vi "PicoScope3000aAdvancedTriggerSettingsV2.vi"(0 "error in":errorcluster, 1 "handle in":i16, 3 "Trigger Conditions":T6 {"Condition Logic" items=["AND", "OR", "XOR"]}, 4 "Trigger Delay":u32, 5 "Auto Trigger (ms)":i32=1000, 6 "Channel A Trigger Properties":T3={"thresholdUpper"=0, "thresholdUpperHysteresis"=5, "thresholdLower"=0, "thresholdLowerHysteresis"=5, "Threshold Mode"=0, "Direction"=2, "Available"=FALSE} {"Direction" items=["Above / Inside", "Below / Outside", "Rising / Enter", "Falling / Exit", "Rising or Falling / Enter or Exit", "Above Lower", "Below Lower", "Rising Lower", "Falling Lower", "Positive Runt", "Negative Runt"]; "Threshold Mode" items=["Level", "Window"]}, 7 "Channel D Trigger Properties":T3={"thresholdUpper"=0, "thresholdUpperHysteresis"=0, "thresholdLower"=0, "thresholdLowerHysteresis"=0, "Threshold Mode"=0, "Direction"=2, "Available"=FALSE} {"Direction" items=["Above / Inside", "Below / Outside", "Rising / Enter", "Falling / Exit", "Rising or Falling / Enter or Exit", "Above Lower", "Below Lower", "Rising Lower", "Falling Lower", "Positive Runt", "Negative Runt"]; "Threshold Mode" items=["Level", "Window"]}, 8 "Channel B Trigger Properties":T3={"thresholdUpper"=0, "thresholdUpperHysteresis"=0, "thresholdLower"=0, "thresholdLowerHysteresis"=0, "Threshold Mode"=0, "Direction"=2, "Available"=FALSE} {"Direction" items=["Above / Inside", "Below / Outside", "Rising / Enter", "Falling / Exit", "Rising or Falling / Enter or Exit", "Above Lower", "Below Lower", "Rising Lower", "Falling Lower", "Positive Runt", "Negative Runt"]; "Threshold Mode" items=["Level", "Window"]}, 10 "Digital Port  0":T2 {"Direction Channel 7" items=["Don't Care", "Low", "High", "Rising", "Falling"]; "Direction Channel 6" items=["Don't Care", "Low", "High", "Rising", "Falling"]; "Direction Channel 5" items=["Don't Care", "Low", "High", "Rising", "Falling"]; "Direction Channel 4" items=["Don't Care", "Low", "High", "Rising", "Falling"]; "Direction Channel 3" items=["Don't Care", "Low", "High", "Rising", "Falling"]; "Direction Channel 2" items=["Don't Care", "Low", "High", "Rising", "Falling"]; "Direction Channel 1" items=["Don't Care", "Low", "High", "Rising", "Falling"]; "Direction Channel 0" items=["Don't Care", "Low", "High", "Rising", "Falling"]}, 11 "Ext. Trigger Properties":T3={"thresholdUpper"=0, "thresholdUpperHysteresis"=0, "thresholdLower"=0, "thresholdLowerHysteresis"=0, "Threshold Mode"=0, "Direction"=2, "Available"=FALSE} {"Direction" items=["Above / Inside", "Below / Outside", "Rising / Enter", "Falling / Exit", "Rising or Falling / Enter or Exit", "Above Lower", "Below Lower", "Rising Lower", "Falling Lower", "Positive Runt", "Negative Runt"]; "Threshold Mode" items=["Level", "Window"]}, 12 "Digital Port  1":T1 {"Direction Channel 15" items=["Don't Care", "Low", "High", "Rising", "Falling"]; "Direction Channel 14" items=["Don't Care", "Low", "High", "Rising", "Falling"]; "Direction Channel 13" items=["Don't Care", "Low", "High", "Rising", "Falling"]; "Direction Channel 12" items=["Don't Care", "Low", "High", "Rising", "Falling"]; "Direction Channel 11" items=["Don't Care", "Low", "High", "Rising", "Falling"]; "Direction Channel 10" items=["Don't Care", "Low", "High", "Rising", "Falling"]; "Direction Channel 9" items=["Don't Care", "Low", "High", "Rising", "Falling"]; "Direction Channel 8" items=["Don't Care", "Low", "High", "Rising", "Falling"]}, 13 "Aux. Trigger Properties":T3={"thresholdUpper"=0, "thresholdUpperHysteresis"=0, "thresholdLower"=0, "thresholdLowerHysteresis"=0, "Threshold Mode"=0, "Direction"=2, "Available"=FALSE} {"Direction" items=["Above / Inside", "Below / Outside", "Rising / Enter", "Falling / Exit", "Rising or Falling / Enter or Exit", "Above Lower", "Below Lower", "Rising Lower", "Falling Lower", "Positive Runt", "Negative Runt"]; "Threshold Mode" items=["Level", "Window"]}, 16 "Channel C Trigger Properties":T3={"thresholdUpper"=0, "thresholdUpperHysteresis"=0, "thresholdLower"=0, "thresholdLowerHysteresis"=0, "Threshold Mode"=0, "Direction"=2, "Available"=FALSE} {"Direction" items=["Above / Inside", "Below / Outside", "Rising / Enter", "Falling / Exit", "Rising or Falling / Enter or Exit", "Above Lower", "Below Lower", "Rising Lower", "Falling Lower", "Positive Runt", "Negative Runt"]; "Threshold Mode" items=["Level", "Window"]}, 18 "Pulse Width Qualifier Conditions":T5 {"Condition Logic" items=["AND", "OR", "XOR"]}, 19 "Pulse Width Qualifier Settings":T4={"Direction"=2, "Lower Limit"=0, "Upper Limit"=0, "Pulse Width Type"=0} {"Pulse Width Type" items=["None", "Less Than", "Greater Than", "In Range", "Out of Range"]; "Direction" items=["Rising"=2, "Falling"=3]}) -> (14 "error out":errorcluster, 15 "handle out":i16)   [LabVIEW 2010]
doc: "This VI is an interface for the advanced trigger features of the oscilloscope (a simple trigger can be set using PicoScope3000aSettings.vi, in which case it is not necessary to use this VI)."
uses:
  ps3000a.dll
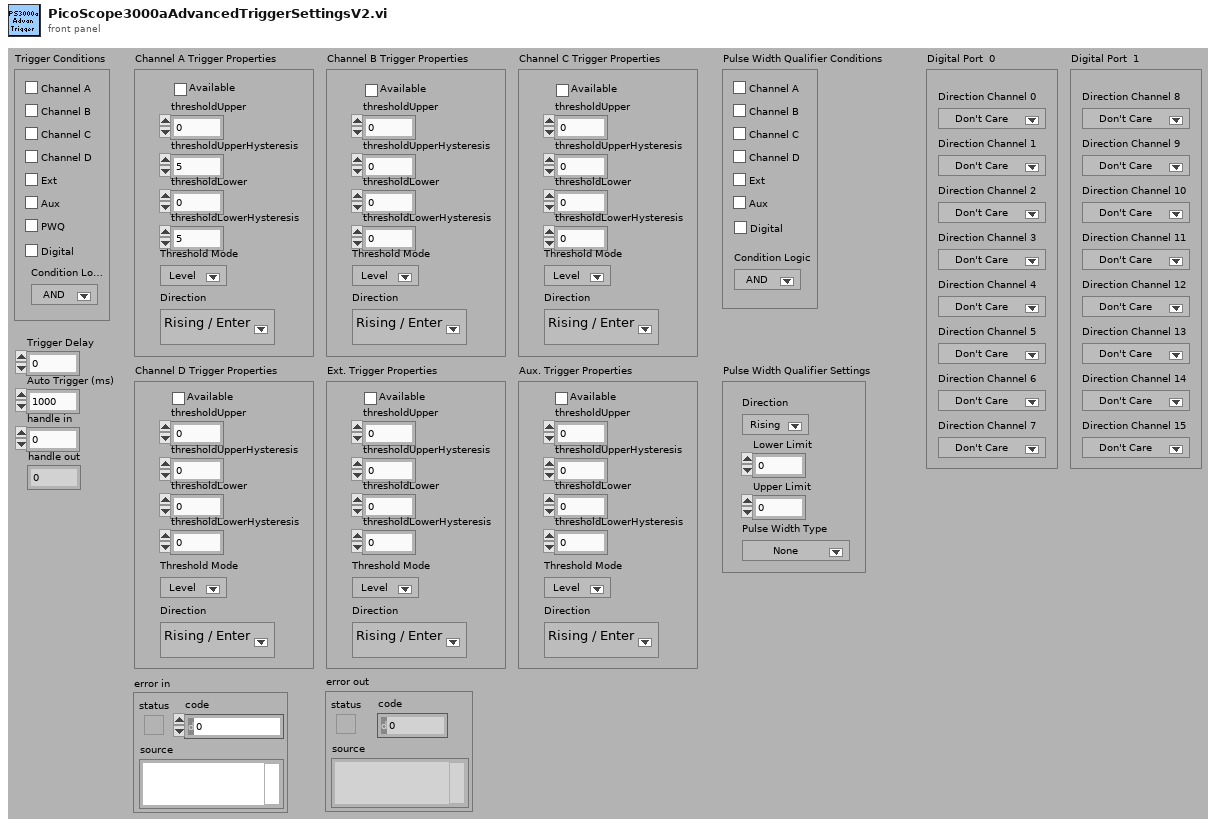
[diagram p1: front panel]
types:
  T1 = cluster{"Direction Channel 8":u16, "Direction Channel 9":u16, "Direction Channel 10":u16, "Direction Channel 11":u16, "Direction Channel 12":u16, "Direction Channel 13":u16, "Direction Channel 14":u16, "Direction Channel 15":u16}
  T2 = cluster{"Direction Channel 0":u16, "Direction Channel 1":u16, "Direction Channel 2":u16, "Direction Channel 3":u16, "Direction Channel 4":u16, "Direction Channel 5":u16, "Direction Channel 6":u16, "Direction Channel 7":u16}
  T3 = cluster{"thresholdUpper":i16, "thresholdUpperHysteresis":u16, "thresholdLower":i16, "thresholdLowerHysteresis":u16, "Threshold Mode":i32, "Direction":i32, "Available":bool}
  T4 = cluster{"Direction":u32, "Lower Limit":u32, "Upper Limit":u32, "Pulse Width Type":u32}
  T5 = cluster{"Channel A":bool, "Channel B":bool, "Channel C":bool, "Channel D":bool, "Aux":bool, "Condition Logic":u16, "Ext":bool, "Digital":bool}
  T6 = cluster{"Channel A":bool, "Channel B":bool, "Channel C":bool, "Channel D":bool, "Aux":bool, "PWQ":bool, "Condition Logic":u16, "Ext":bool, "Digital":bool}
  T7 = cluster{"thresholdUpper":i16, "thresholdUpperHysteresis":u16, "thresholdLower":i16, "thresholdLowerHysteresis":u16, "Threshold Mode":i32, "Direction":i32, "Available":bool}[]
  T8 = cluster{"[0]":u32, "[1]":u32, "[2]":u32, "[3]":u32, "[4]":u32, "[5]":u32, "[6]":u32, "[7]":u32, "[8]":u32}
  T9 = cluster{"status":bool, "code":u32, "source":string}
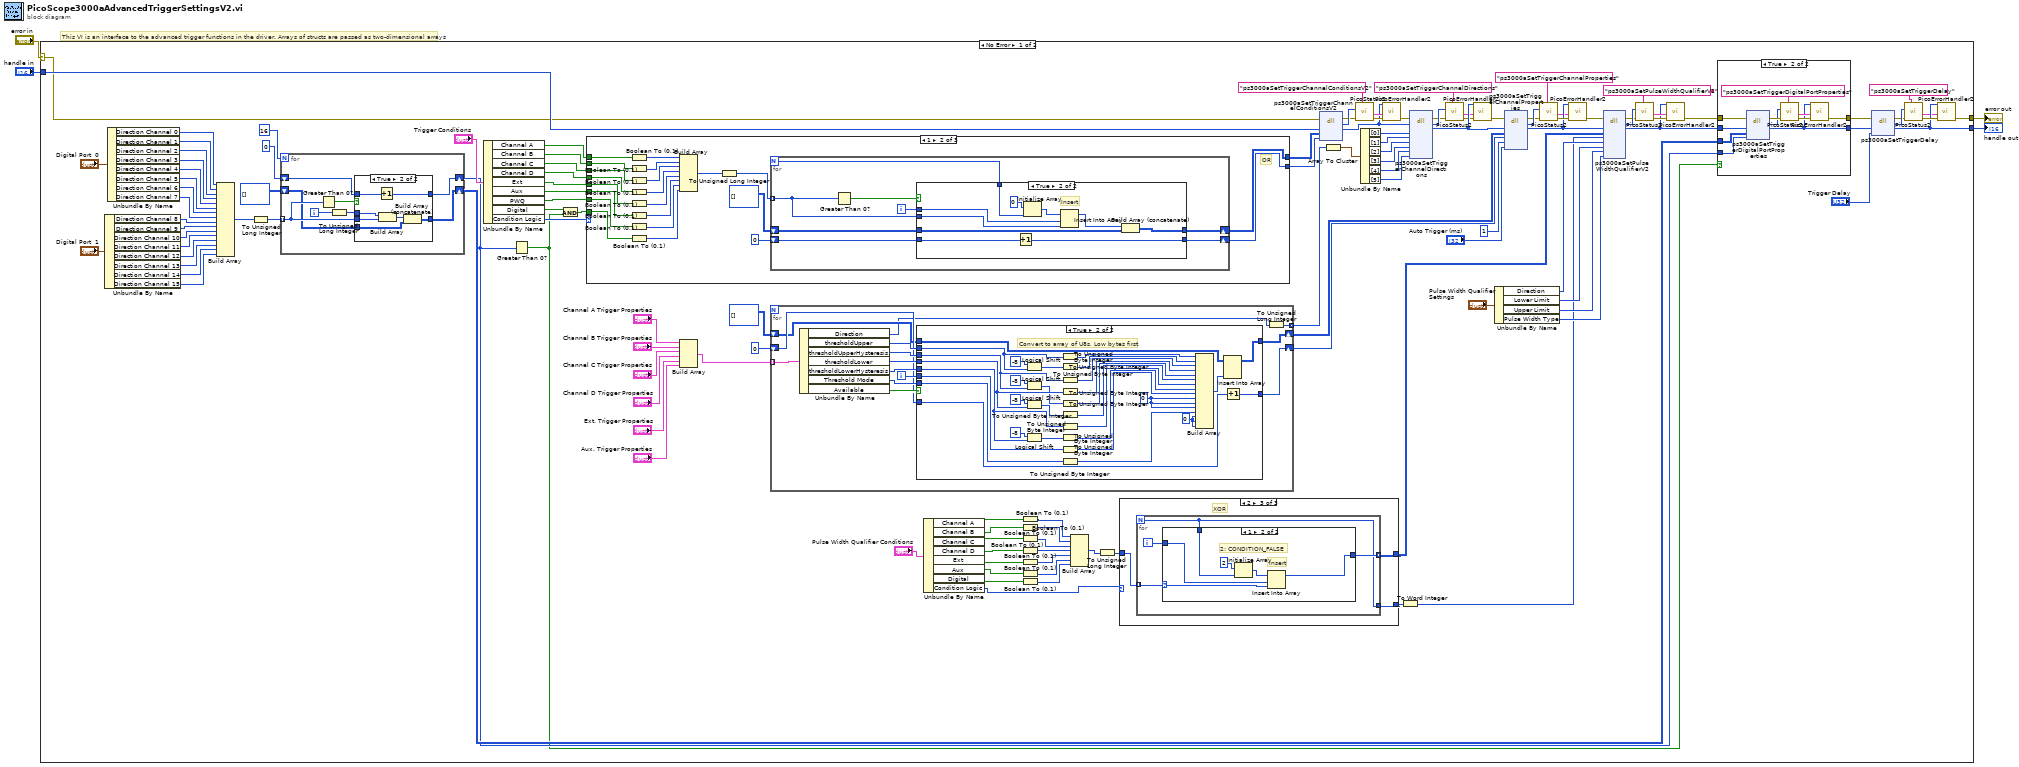
[diagram p0: block diagram]
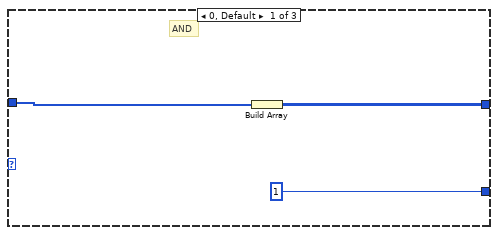
[diagram p2: hidden frame]
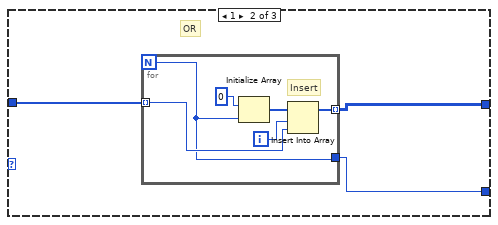
[diagram p3: hidden frame]
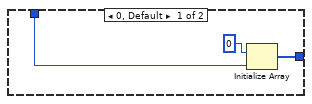
[diagram p4: hidden frame]
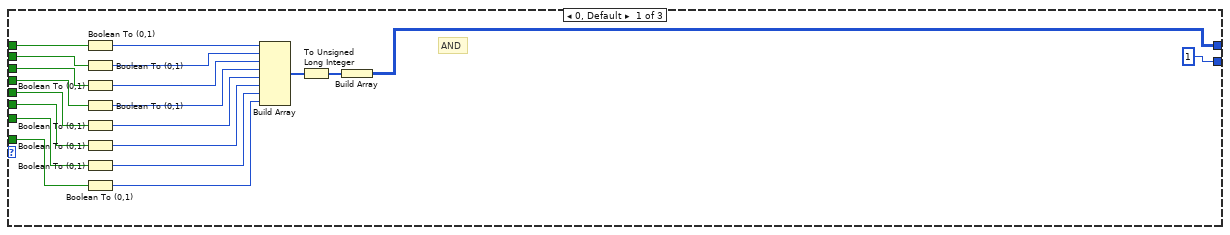
[diagram p8: hidden frame]
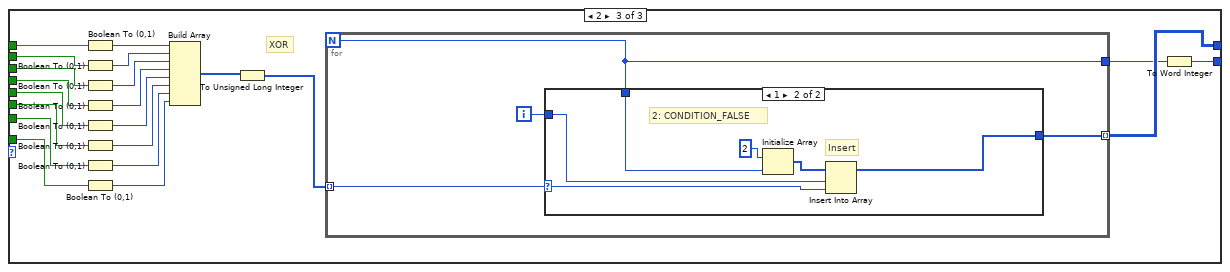
[diagram p10: hidden frame]
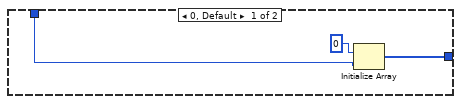
[diagram p11: hidden frame]
diagram:
  # "This VI is an interface to the advanced trigger functions in the driver. Arrays of structs are passed as two-dimensional arrays"
  n1 = case shown="No Error" "error in" {
    selector: "error in" -> [w100 w332]
    tunnel: "handle in" -> [w104 w333]
    tunnel: [w43 w333] -> w2
    tunnel: [w44 w332] -> w1
    frame No Error {
      n2 = Unbundle By Name("Digital Port  1") -> ("Direction Channel 8"=w66:u16, "Direction Channel 9"=w65:u16, "Direction Channel 10"=w64:u16, "Direction Channel 11"=w63:u16, "Direction Channel 12"=w62:u16, "Direction Channel 13"=w61:u16, "Direction Channel 14"=w60:u16, "Direction Channel 15"=w59:u16)
      n3 = Unbundle By Name("Digital Port  0") -> ("Direction Channel 0"=w78:u16, "Direction Channel 1"=w77:u16, "Direction Channel 2"=w76:u16, "Direction Channel 3"=w75:u16, "Direction Channel 4"=w74:u16, "Direction Channel 5"=w73:u16, "Direction Channel 6"=w72:u16, "Direction Channel 7"=w71:u16)
      n4 = Build Array(w78, w77, w76, w75, w74, w73, w72, w71, w66, w65, w64, w63, w62, w61, w60, w59) -> (w38:u16[])
      n5 = To Unsigned Long Integer(number=w38) -> (unsigned 32bit integer=w39:u32[])
      n6 = for {
        N: 16 -> [_]
        tunnel: w39 -> [w178] mode=indexing
        shift-right: [w177] -> w56
        shift-left: u32[][] [] -> [w176]
        shift-right: [w175] -> w53
        shift-left: i16 0 -> [w174]
        i -> [w172]
        n7 = Greater Than 0?(x=w178) -> (x > 0?=w179:bool)
        n8 = To Unsigned Long Integer(number=w172) -> (unsigned 32bit integer=w173:u32)
        n9 = case shown="True" w179 {
          tunnel: w173 -> [_ w188]
          tunnel: w178 -> [_ w187]
          tunnel: [w181 w185] -> w177
          tunnel: w176 -> [w181 w184]
          tunnel: [w180 w183] -> w175
          tunnel: w174 -> [w180 w182]
          frame False {
          }
          frame True {
            n10 = Increment(x=w182) -> (x+1=w183:i16)
            n11 = Build Array(w188, w187) -> (w186:u32[])
            n12 = Build Array (concatenate)(w186, w184) -> (w185:u32[][])
          }
        }
      }
      n13 = Unbundle By Name("Trigger Conditions") -> ("Channel A"=w85:bool, "Channel B"=w84:bool, "Channel C"=w83:bool, "Channel D"=w82:bool, "Ext"=w81:bool, "Aux"=w80:bool, "PWQ"=w79:bool, "Digital"=w55:bool, "Condition Logic"=w86:u16)
      n14 = Greater Than 0?(x=w53) -> (x > 0?=w52:bool)
      n15 = And(x=w55, y=w52) -> (x .and. y?=w54:bool)
      n16 = case shown="1" w86 {
        tunnel: [w255 w270 w311] -> w128
        tunnel: [i16 1 w268 w298] -> w127
        tunnel: w85 -> [w253 w265 w309]
        tunnel: w84 -> [w252 w264 w308]
        tunnel: w83 -> [w251 w263 w307]
        tunnel: w82 -> [w250 w262 w306]
        tunnel: w81 -> [w249 w261 w305]
        tunnel: w80 -> [w248 w260 w304]
        tunnel: w79 -> [w247 w259 w303]
        tunnel: w54 -> [w246 w258 w302]
        frame 0, Default {
          # "AND"
          n17 = Boolean To (0,1)(Boolean=w253) -> (0, 1=w245:i16)
          n18 = Boolean To (0,1)(Boolean=w252) -> (0, 1=w244:i16)
          n19 = Boolean To (0,1)(Boolean=w251) -> (0, 1=w238:i16)
          n20 = Boolean To (0,1)(Boolean=w250) -> (0, 1=w239:i16)
          n21 = Boolean To (0,1)(Boolean=w249) -> (0, 1=w240:i16)
          n22 = Boolean To (0,1)(Boolean=w248) -> (0, 1=w241:i16)
          n23 = Boolean To (0,1)(Boolean=w247) -> (0, 1=w242:i16)
          n24 = Boolean To (0,1)(Boolean=w246) -> (0, 1=w243:i16)
          n25 = Build Array(w245, w244, w238, w239, w240, w241, w242, w243) -> (w237:i16[])
          n26 = To Unsigned Long Integer(number=w237) -> (unsigned 32bit integer=w236:u32[])
          n27 = Build Array(w236) -> (w255:u32[][])
        }
        frame 1 {
          # "OR"
          n28 = Boolean To (0,1)(Boolean=w265) -> (0, 1=w271:i16)
          n29 = Boolean To (0,1)(Boolean=w264) -> (0, 1=w272:i16)
          n30 = Boolean To (0,1)(Boolean=w263) -> (0, 1=w273:i16)
          n31 = Boolean To (0,1)(Boolean=w262) -> (0, 1=w274:i16)
          n32 = Boolean To (0,1)(Boolean=w261) -> (0, 1=w275:i16)
          n33 = Boolean To (0,1)(Boolean=w260) -> (0, 1=w276:i16)
          n34 = Boolean To (0,1)(Boolean=w259) -> (0, 1=w277:i16)
          n35 = Boolean To (0,1)(Boolean=w258) -> (0, 1=w266:i16)
          n36 = Build Array(w271, w272, w273, w274, w275, w276, w277, w266) -> (w257:i16[])
          n37 = To Unsigned Long Integer(number=w257) -> (unsigned 32bit integer=w256:u32[])
          n38 = for {
            N -> [w278]
            tunnel: w256 -> [w282] mode=indexing
            shift-right: [w281] -> w270
            shift-left: u32[][] [] -> [w285]
            shift-right: [w279] -> w268
            shift-left: i16 0 -> [w280]
            i -> [w284]
            n39 = Greater Than 0?(x=w282) -> (x > 0?=w283:bool)
            n40 = case shown="True" w283 {
              tunnel: w285 -> [w287 w291]
              tunnel: w284 -> [_ w295]
              tunnel: w282 -> [_ w294]
              tunnel: [w287 w293] -> w281
              tunnel: w280 -> [w286 w290]
              tunnel: [w286 w289] -> w279
              tunnel: w278 -> [_ w288]
              frame False {
              }
              frame True {
                # "Insert"
                n41 = Increment(x=w290) -> (x+1=w289:i16)
                n42 = Initialize Array(u32 0 ("element"), w288) -> (w296:u32[])
                n43 = Insert Into Array(array=w296, index=w295, new element=w294) -> (w292:u32[])
                n44 = Build Array (concatenate)(w292, w291) -> (w293:u32[][])
              }
            }
          }
        }
        frame 2 {
          # "XOR"
          n45 = Boolean To (0,1)(Boolean=w309) -> (0, 1=w312:i16)
          n46 = Boolean To (0,1)(Boolean=w308) -> (0, 1=w313:i16)
          n47 = Boolean To (0,1)(Boolean=w307) -> (0, 1=w314:i16)
          n48 = Boolean To (0,1)(Boolean=w306) -> (0, 1=w315:i16)
          n49 = Boolean To (0,1)(Boolean=w305) -> (0, 1=w316:i16)
          n50 = Boolean To (0,1)(Boolean=w304) -> (0, 1=w317:i16)
          n51 = Boolean To (0,1)(Boolean=w303) -> (0, 1=w318:i16)
          n52 = Boolean To (0,1)(Boolean=w302) -> (0, 1=w310:i16)
          n53 = Build Array(w312, w313, w314, w315, w316, w317, w318, w310) -> (w301:i16[])
          n54 = To Unsigned Long Integer(number=w301) -> (unsigned 32bit integer=w300:u32[])
          n55 = for {
            N -> [w319]
            tunnel: w300 -> [w320] mode=indexing
            tunnel: [w322] -> w311 mode=indexing
            tunnel: [w319] -> w299
            i -> [w321]
            n56 = case shown="1" w320 {
              selector: w320 -> [_ w328]
              tunnel: [w324 w329] -> w322
              tunnel: w321 -> [_ w327]
              tunnel: w319 -> [w323 w326]
              frame 0, Default {
                n57 = Initialize Array(u32 0 ("element"), w323) -> (w324:u32[])
              }
              frame 1 {
                # "2: CONDITION_FALSE"
                # "Insert"
                n58 = Initialize Array(u32 2 ("element"), w326) -> (w330:u32[])
                n59 = Insert Into Array(array=w330, index=w327, new element=w328) -> (w329:u32[])
              }
            }
          }
          n60 = To Word Integer(number=w299) -> (16bit integer=w298:i16)
        }
      }
      n61 = Build Array("Channel A Trigger Properties", "Channel B Trigger Properties", "Channel C Trigger Properties", "Channel D Trigger Properties", "Ext. Trigger Properties", "Aux. Trigger Properties") -> (w125:T7)
      n62 = for {
        tunnel: w125 -> [w197] mode=indexing
        tunnel: [w190] -> w124 mode=indexing
        shift-right: [w194] -> w89
        shift-left: i16 0 -> [w193]
        shift-right: [w191] -> w87
        shift-left: u8[][] [] -> [w192]
        i -> [w195]
        n63 = Unbundle By Name(w197) -> ("Direction"=w189:i32, "thresholdUpper"=w202:i16, "thresholdUpperHysteresis"=w201:u16, "thresholdLower"=w200:i16, "thresholdLowerHysteresis"=w199:u16, "Threshold Mode"=w198:i32, "Available"=w196:bool)
        n64 = case shown="True" w196 {
          tunnel: w202 -> [_ w234]
          tunnel: w201 -> [_ w226]
          tunnel: w200 -> [_ w225]
          tunnel: w199 -> [_ w224]
          tunnel: w198 -> [_ w215]
          tunnel: w195 -> [_ w210]
          tunnel: [w204 w209] -> w194
          tunnel: w193 -> [w204 w208]
          tunnel: [w203 w206] -> w191
          tunnel: w192 -> [w203 w205]
          frame False {
          }
          frame True {
            w213 = u8 0 ("element")
            w214 = u8 0 ("element")
            # "Convert to array of U8s, Low bytes first"
            n65 = Logical Shift(y=i16 -8, x=w234) -> (x << y=w233:i16)
            n66 = Logical Shift(y=i16 -8, x=w226) -> (x << y=w232:u16)
            n67 = Logical Shift(y=i16 -8, x=w225) -> (x << y=w229:i16)
            n68 = Logical Shift(y=i16 -8, x=w224) -> (x << y=w228:u16)
            n69 = To Unsigned Byte Integer(number=w234) -> (unsigned 8bit integer=w223:u8)
            n70 = To Unsigned Byte Integer(number=w233) -> (unsigned 8bit integer=w222:u8)
            n71 = To Unsigned Byte Integer(number=w226) -> (unsigned 8bit integer=w221:u8)
            n72 = To Unsigned Byte Integer(number=w232) -> (unsigned 8bit integer=w220:u8)
            n73 = To Unsigned Byte Integer(number=w225) -> (unsigned 8bit integer=w219:u8)
            n74 = To Unsigned Byte Integer(number=w229) -> (unsigned 8bit integer=w218:u8)
            n75 = To Unsigned Byte Integer(number=w224) -> (unsigned 8bit integer=w217:u8)
            n76 = To Unsigned Byte Integer(number=w228) -> (unsigned 8bit integer=w216:u8)
            n77 = To Unsigned Byte Integer(number=w210) -> (unsigned 8bit integer=w211:u8)
            n78 = To Unsigned Byte Integer(number=w215) -> (unsigned 8bit integer=w212:u8)
            n79 = Build Array(w223, w222, w221, w220, w219, w218, w217, w216, w211, w214, w214, w214, w212, w213, w213, w213) -> (w207:u8[])
            n80 = Insert Into Array(array=w205, new element=w207) -> (w206:u8[][])  [unwired: 2 in]
            n81 = Increment(x=w208) -> (x+1=w209:i16)
          }
        }
        n82 = To Unsigned Long Integer(number=w189) -> (unsigned 32bit integer=w190:u32)
      }
      n83 = Unbundle By Name("Pulse Width Qualifier Conditions") -> ("Channel A"=w21:bool, "Channel B"=w22:bool, "Channel C"=w23:bool, "Channel D"=w24:bool, "Ext"=w25:bool, "Aux"=w26:bool, "Digital"=w27:bool, "Condition Logic"=w28:u16)
      n84 = Boolean To (0,1)(Boolean=w21) -> (0, 1=w20:i16)
      n85 = Boolean To (0,1)(Boolean=w22) -> (0, 1=w33:i16)
      n86 = Boolean To (0,1)(Boolean=w23) -> (0, 1=w34:i16)
      n87 = Boolean To (0,1)(Boolean=w24) -> (0, 1=w35:i16)
      n88 = Boolean To (0,1)(Boolean=w25) -> (0, 1=w36:i16)
      n89 = Boolean To (0,1)(Boolean=w26) -> (0, 1=w37:i16)
      n90 = Boolean To (0,1)(Boolean=w27) -> (0, 1=w32:i16)
      n91 = Build Array(w20, w33, w34, w35, w36, w37, w32) -> (w31:i16[])
      n92 = To Unsigned Long Integer(number=w31) -> (unsigned 32bit integer=w30:u32[])
      n93 = case shown="2" w28 {
        tunnel: [w133 w136 w145] -> w18
        tunnel: [u32 1 w134 w144] -> w29
        tunnel: w30 -> [w131 w135 w143]
        frame 0, Default {
          # "AND"
          n94 = Build Array(w131) -> (w133:u32[][])
        }
        frame 1 {
          # "OR"
          n95 = for {
            N -> [w137]
            tunnel: w135 -> [w139] mode=indexing
            tunnel: [w138] -> w136 mode=indexing
            tunnel: [w137] -> w134
            i -> [w140]
            # "Insert"
            n96 = Initialize Array(u32 0 ("element"), w137) -> (w141:u32[])
            n97 = Insert Into Array(array=w141, index=w140, new element=w139) -> (w138:u32[])
          }
        }
        frame 2 {
          # "XOR"
          n98 = for {
            N -> [w146]
            tunnel: w143 -> [w149] mode=indexing
            tunnel: [w147] -> w145 mode=indexing
            tunnel: [w146] -> w144
            i -> [w148]
            n99 = case shown="1" w149 {
              selector: w149 -> [_ w155]
              tunnel: [w151 w156] -> w147
              tunnel: w148 -> [_ w154]
              tunnel: w146 -> [w150 w153]
              frame 0, Default {
                n100 = Initialize Array(u32 0 ("element"), w150) -> (w151:u32[])
              }
              frame 1 {
                # "2: CONDITION_FALSE"
                # "Insert"
                n101 = Initialize Array(u32 2 ("element"), w153) -> (w157:u32[])
                n102 = Insert Into Array(array=w157, index=w154, new element=w155) -> (w156:u32[])
              }
            }
          }
        }
      }
      n103 = dll-call lib="ps3000a.dll" fn="ps3000aSetTriggerChannelConditionsV2" ("ps3000.dll:_ps3000_open_unit@0")(error in=w100, "handle"=w104, "conditions"=w128, "nConditions"=w127) -> (error out=w102:errorcluster, "PICO_STATUS"=w103:u32, "handle"=w14:i16)  [unwired: 4 in, 1 out]
      n104 = Array To Cluster(array=w124) -> (cluster=w123:T8)
      n105 = call "PicoStatus2.vi"("PICO source"="ps3000aSetTriggerChannelConditionsV2" ("source"), "Error in"=w102, "PICO STATUS"=w103) -> ("error out"=w17:errorcluster, "PICO_STATUS out"=w16:T9)  [unwired: 5 in]
      n106 = Unbundle By Name(w123) -> ("[0]"=w122:u32, "[1]"=w121:u32, "[2]"=w120:u32, "[3]"=w119:u32, "[4]"=w118:u32, "[5]"=w117:u32)
      n107 = call "PicoErrorHandler2.vi"("error in (no error)"=w17, "PICO_STATUS in"=w16, "handle In"=w14) -> ("error out"=w15:errorcluster)  [unwired: 8 in]
      n108 = To Word Integer(number=w29) -> (16bit integer=w19:i16)
      n109 = dll-call lib="ps3000a.dll" fn="ps3000aSetTriggerChannelDirections" ("ps3000.dll:_ps3000_open_unit@0")(error in=w15, "handle"=w14, "channelA"=w122, "channelB"=w121, "channelC"=w120, "channelD"=w119, "ext"=w118, "aux"=w117) -> (error out=w98:errorcluster, "PICO_STATUS"=w99:u32, "handle"=w50:i16)  [unwired: 8 in, 1 out]
      n110 = call "PicoStatus2.vi"("PICO source"="ps3000aSetTriggerChannelDirections" ("source"), "Error in"=w98, "PICO STATUS"=w99) -> ("error out"=w49:errorcluster, "PICO_STATUS out"=w13:T9)  [unwired: 5 in]
      n111 = call "PicoErrorHandler2.vi"("error in (no error)"=w49, "PICO_STATUS in"=w13, "handle In"=w50) -> ("error out"=w51:errorcluster)  [unwired: 8 in]
      n112 = Unbundle By Name("Pulse Width Qualifier Settings") -> ("Direction"=w113:u32, "Lower Limit"=w112:u32, "Upper Limit"=w111:u32, "Pulse Width Type"=w110:u32)
      n113 = dll-call lib="ps3000a.dll" fn="ps3000aSetTriggerChannelProperties" ("ps3000.dll:_ps3000_open_unit@0")(error in=w51, "handle"=w50, "channelProperties"=w87, "nChannelProperties"=w89, "auxOutputEnable"=i16 1, "autoTriggerMilliseconds"="Auto Trigger (ms)") -> (error out=w96:errorcluster, "PICO_STATUS"=w97:u32, "handle"=w40:i16)  [unwired: 6 in, 1 out]
      n114 = call "PicoStatus2.vi"("PICO source"="ps3000aSetTriggerChannelProperties" ("source"), "Error in"=w96, "PICO STATUS"=w97) -> ("error out"=w41:errorcluster, "PICO_STATUS out"=w12:T9)  [unwired: 5 in]
      n115 = call "PicoErrorHandler2.vi"("error in (no error)"=w41, "PICO_STATUS in"=w12, "handle In"=w40) -> ("error out"=w42:errorcluster)  [unwired: 8 in]
      n116 = dll-call lib="ps3000a.dll" fn="ps3000aSetPulseWidthQualifierV2" ("ps3000.dll:_ps3000_open_unit@0")(error in=w42, "handle"=w40, "conditions"=w18, "nConditions"=w19, "direction"=w113, "lower"=w112, "upper"=w111, "type"=w110) -> (error out=w47:errorcluster, "PICO_STATUS"=w48:u32, "handle"=w9:i16)  [unwired: 8 in, 1 out]
      n117 = call "PicoStatus2.vi"("PICO source"="ps3000aSetPulseWidthQualifierV2" ("source"), "Error in"=w47, "PICO STATUS"=w48) -> ("error out"=w11:errorcluster, "PICO_STATUS out"=w10:T9)  [unwired: 5 in]
      n118 = call "PicoErrorHandler2.vi"("error in (no error)"=w11, "PICO_STATUS in"=w10, "handle In"=w9) -> ("error out"=w8:errorcluster)  [unwired: 8 in]
      n119 = case shown="True" w52 {
        tunnel: w8 -> [w159 w170]
        tunnel: w9 -> [w160 w169]
        tunnel: [w160 w162] -> w6
        tunnel: w53 -> [_ w165]
        tunnel: w56 -> [_ w166]
        tunnel: [w159 w161] -> w7
        frame False {
        }
        frame True {
          n120 = dll-call lib="ps3000a.dll" fn="ps3000aSetTriggerDigitalPortProperties"(error in=w170, "handle"=w169, "digitalDirections"=w166, "nDigitalDirections"=w165) -> (error out=w168:errorcluster, "PICO_STATUS"=w167:u32, "handle"=w162:i16)  [unwired: 4 in, 1 out]
          n121 = call "PicoStatus2.vi"("PICO source"="ps3000aSetTriggerDigitalPortProperties" ("source"), "Error in"=w168, "PICO STATUS"=w167) -> ("error out"=w164:errorcluster, "PICO_STATUS out"=w163:T9)  [unwired: 5 in]
          n122 = call "PicoErrorHandler2.vi"("error in (no error)"=w164, "PICO_STATUS in"=w163, "handle In"=w162) -> ("error out"=w161:errorcluster)  [unwired: 8 in]
        }
      }
      n123 = dll-call lib="ps3000a.dll" fn="ps3000aSetTriggerDelay" ("ps3000.dll:_ps3000_open_unit@0")(error in=w7, "handle"=w6, "delay"="Trigger Delay") -> (error out=w94:errorcluster, "PICO_STATUS"=w95:u32, "handle"=w43:i16)  [unwired: 3 in, 1 out]
      n124 = call "PicoStatus2.vi"("PICO source"="ps3000aSetTriggerDelay" ("source"), "Error in"=w94, "PICO STATUS"=w95) -> ("error out"=w45:errorcluster, "PICO_STATUS out"=w5:T9)  [unwired: 5 in]
      n125 = call "PicoErrorHandler2.vi"("error in (no error)"=w45, "PICO_STATUS in"=w5, "handle In"=w43) -> ("error out"=w44:errorcluster)  [unwired: 8 in]
    }
    frame Error {
    }
  }
  "handle out" <- w2
  "error out" <- w1
